vi "Tester.vi"() -> ()   [LabVIEW 2023]
uses:
  <vilib>/Utility/libraryn.llb/Get File Extension.vi
panel:
  out "Array 2":string[](array[string])
  out "Array":string[](array[string])
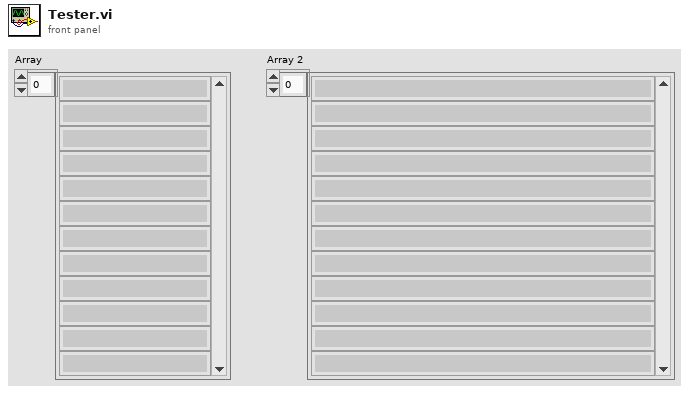
[diagram p1: front panel]
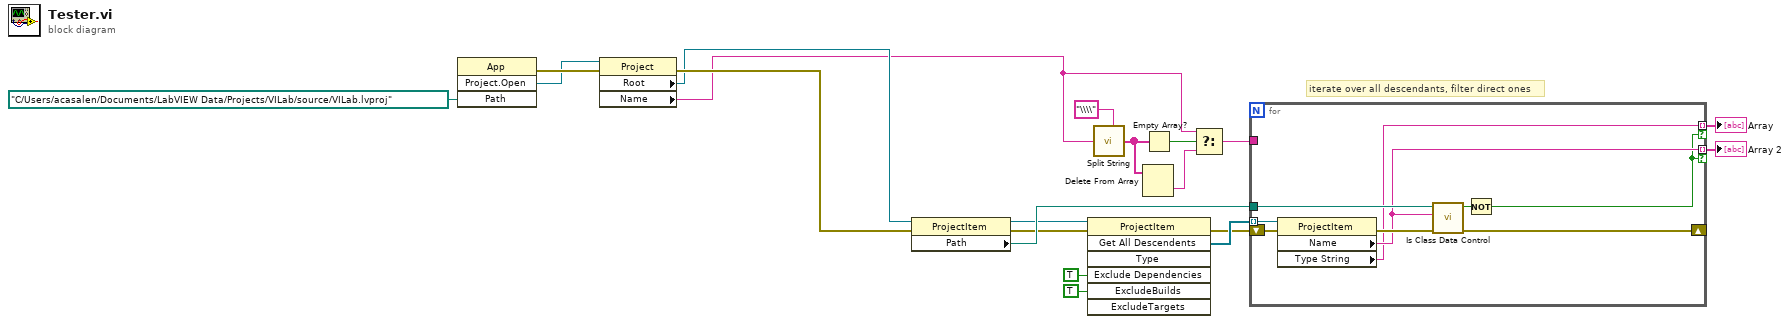
[diagram p0: block diagram]
diagram:
  # "iterate over all descendants, filter direct ones"
  n1 = invoke class="App" method="Project.Open"("Path"=path "C:/Users/acasalen/Documents/LabVIEW Data/Projects/VILab/source/VILab.lvproj") -> (error out=w19:errorcluster, "Project:Open"=w18:refnum<vi>)  [unwired: 3 in, 2 out]
  n2 = property class="Project"(reference=w18, error in=w19) -> (error out=w20:errorcluster, "Root"=w17:refnum<vi>, "Name"=w16:string)  [unwired: 1 out]
  n3 = property class="ProjectItem"(reference=w17, error in=w20) -> (reference out=w14:refnum<vi>, error out=w5:errorcluster, "Path"=w15:path)
  n4 = invoke class="ProjectItem" method="Get All Descendents"(reference=w14, error in=w5, "Exclude Dependencies"=TRUE ("ExcludeDependencies"), "ExcludeBuilds"=TRUE) -> (error out=w4:errorcluster, "All Descendents"=w6:refnum<vi>[])  [unwired: 3 in, 5 out]
  n5 = call <vilib>:"Split String.vi"("Split Pattern"="\\\\", "Input String"=w16) -> ("Split String"=w11:string[])  [unwired: 5 in]
  n6 = Delete From Array(array=w11) -> (deleted portion=w12:string)  [unwired: 2 in, 1 out]
  n7 = Empty Array?(array=w11) -> (empty?=w10:bool)
  n8 = Select(t=w16, s=w10, f=w12) -> (s? t:f=w13:string)
  n9 = for {
    tunnel: w6 -> [w26] mode=indexing
    tunnel: w13 -> [_]
    tunnel: [w23] -> w2 mode=indexing if=w21
    shift-right: [w27] -> _
    shift-left: w4 -> [w29]
    tunnel: w15 -> [w24]
    tunnel: [w22] -> w3 mode=indexing if=w21
    n10 = property class="ProjectItem"(reference=w26, error in=w29) -> (error out=w28:errorcluster, "Name"=w23:string, "Type String"=w22:string)  [unwired: 1 out]
    n11 = call "Is Class Data Control.vi"("error in (no error)"=w28, "Item Name"=w23, "Path"=w24) -> ("error out"=w27:errorcluster, "Is Class Data Control?"=w25:bool)  [unwired: 7 in]
    n12 = Not(x=w25) -> (.not. x?=w21:bool)
  }
  "Array" <- w3
  "Array 2" <- w2
